vi "Stop.vi"(6 "Busy":refnum<vi>, 8 "error in (no error)":errorcluster, 11 "Controlador in":refnum<class "Controlador.lvclass">) -> (0 "error out":errorcluster, 2 "String":string, 3 "Controlador out":refnum<class "Controlador.lvclass">)   [LabVIEW 2011, in "Controlador.lvclass"]
uses:
  Controlador.lvclass
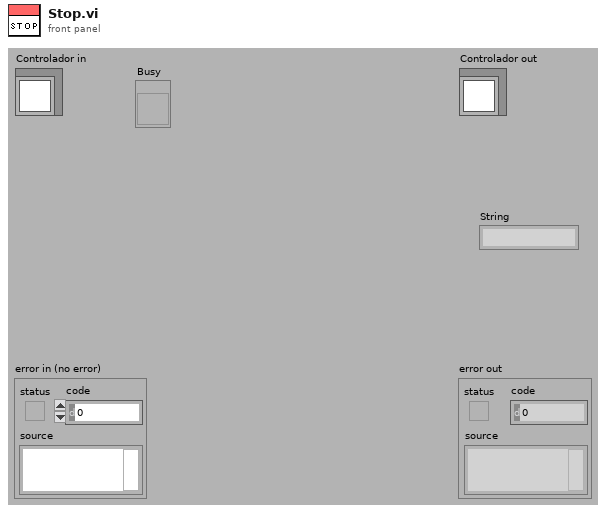
[diagram p1: front panel]
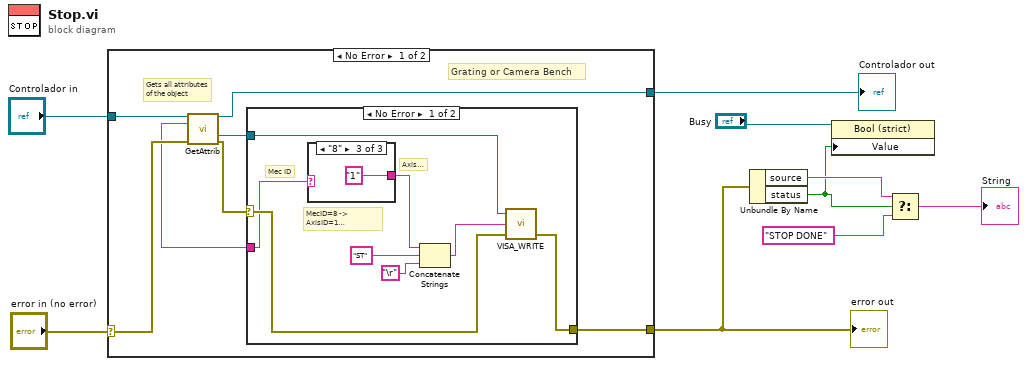
[diagram p0: block diagram]
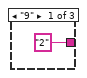
[diagram p2: hidden frame]
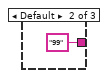
[diagram p3: hidden frame]
diagram:
  n1 = case shown="No Error" "error in (no error)" {
    selector: "error in (no error)" -> [w16 w29]
    tunnel: "Controlador in" -> [w15 w30]
    tunnel: [w12 w30] -> w8
    tunnel: [w10 w29] -> w5
    frame No Error {
      # "Gets all attributes \nof the object"
      # "Grating or Camera Bench"
      n2 = call "GetAttrib.vi"("Device in"=w15, "error in (no error)"=w16) -> ("Device out"=w12:refnum<class "Controlador.lvclass">, "Mec ID"=w13:string, "VISA Mec"=w14:refnum<visa-resource-name>, "error out"=w11:errorcluster)  [unwired: 10 out]
      n3 = case shown="No Error" w11 {
        selector: w11 -> [w19 w28]
        tunnel: [w21 w28] -> w10
        tunnel: w14 -> [w20 _]
        tunnel: w13 -> [w18 _]
        frame No Error {
          # "MecID=8 -> AxisID=1\nMecID=9 -> AxisID=2"
          # "Axis ID"
          # "Mec ID"
          n4 = case shown="\"8\"" w18 {
            tunnel: ["2" "99" "1"] -> w17
            frame "9" {
            }
            frame Default {
            }
            frame "8" {
            }
          }
          n5 = Concatenate Strings(w17, "ST" ("write buffer"), "\r") -> (w22:string)
          n6 = call "VISA_WRITE.vi"("error in (no error)"=w19, "write buffer"=w22, "VISA resource name"=w20) -> ("error out"=w21:errorcluster)  [unwired: 2 out]
        }
        frame Error {
        }
      }
    }
    frame Error {
    }
  }
  "error out" <- w5
  "Controlador out" <- w8
  n7 = Unbundle By Name(w5) -> ("source"=w6:string, "status"=w1:bool)
  n8 = property class="Bool (strict)"(reference="Busy", "Value"=w1) -> ()  [unwired: 1 in, 2 out]
  n9 = Select(t=w6, s=w1, f="STOP DONE" ("string")) -> (s? t:f=→"String":string)
